vi "4a - Write global.vi"() -> ()   [LabVIEW 2010]
uses:
  My Globals.vi
panel:
  in  "start":bool
  out "Chart 1":dbl(graph)
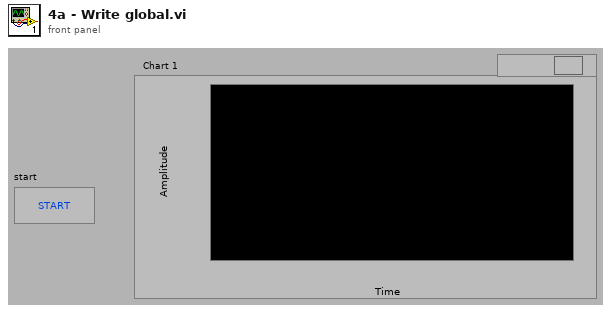
[diagram p1: front panel]
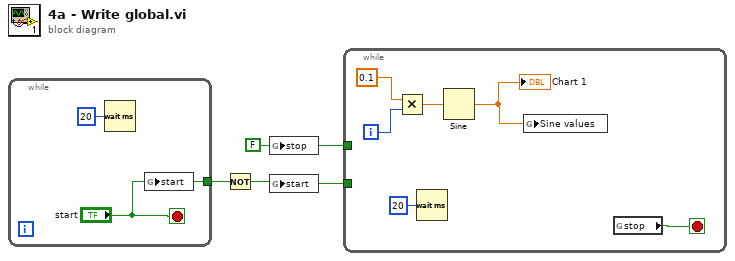
[diagram p0: block diagram]
diagram:
  w1 = FALSE ("stop")
  n1 = while {
    tunnel: ["start"] -> w3
    stop <- "start" stop-if-true
    n2 = Wait (ms)(milliseconds to wait=u32 20) -> ()  [unwired: 1 out]
    n3 = global write "My Globals.vi" "start"("start") -> ()
  }
  n4 = Not(x=w3) -> (.not. x?=w2:bool)
  n5 = global write "My Globals.vi" "stop"(w1) -> ()
  n6 = global write "My Globals.vi" "start"(w2) -> ()
  n7 = while {
    tunnel: w2 -> [_]
    tunnel: w1 -> [_]
    i -> [w9]
    stop <- w7 stop-if-true
    n8 = Multiply(x=0.1, y=w9) -> (x*y=w8:dbl)
    n9 = Wait (ms)(milliseconds to wait=u32 20) -> ()  [unwired: 1 out]
    n10 = Sine(x=w8) -> (sin(x)=w6:dbl)
    "Chart 1" <- w6
    n11 = global write "My Globals.vi" "Sine values"(w6) -> ()
    n12 = global read "My Globals.vi" "stop"() -> (w7:bool)
  }
